vi "GT Get Laser On Time.vi"(8 "error in (no error)":errorcluster caption="错误输入（无错误）", 9 "pTime":u32, 10 "channel":i16, 11 "cardNum":i16) -> (0 "error out":errorcluster caption="错误输出", 1 "pTime out":u32, 3 "function return":i16)   [LabVIEW 2014, in "gts.lvlib"]
doc: "GT_API GT_GetLaserOnTime(short cardNum,short channel,unsigned long *pTime);"
uses:
  gts.lvlib
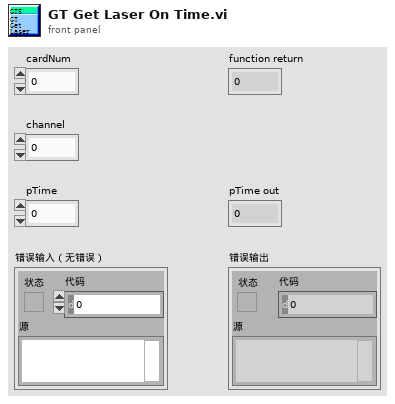
[diagram p1: front panel]
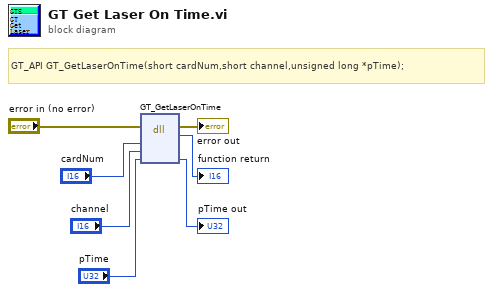
[diagram p0: block diagram]
diagram:
  # "GT_API GT_GetLaserOnTime(short cardNum,short channel,unsigned long *pTime);"
  n1 = dll-call lib="PTH2habs D固高科技资料GTS控制卡GTS卡18年上半年资料dllVC32bit\nmulti_cardgts.*" fn="GT_GetLaserOnTime"(error in="error in (no error)", "cardNum"="cardNum", "channel"="channel", "pTime"="pTime") -> (error out=→"error out":errorcluster, →"function return":i16, "pTime"=→"pTime out":u32)  [unwired: 4 in, 1 out]
